vi "PWM Read Duty.vi"(7 "GPIO #":T1=-1, 8 "error in (no error)":errorcluster, 11 "Session in":refnum<class "Session.lvclass">) -> (0 "error out":errorcluster, 2 "Duty % (0-1)":sgl, 3 "Session out":refnum<class "Session.lvclass">)   [LabVIEW 2024, in "CTI.lvlib" / "Session.lvclass"]
doc: "Returns the current duty cycle (as a range from 0.0 to 1.0) of the PWM output. 0 means the output is completely off while 1 is completely on. Varying the duty cycle can be used for operations like controlling the brightness of an LED."
uses:
  Session.lvclass
  GPIO Number.ctl
  DeviceComms/DeviceComms.lvclass
  CTI.lvlib
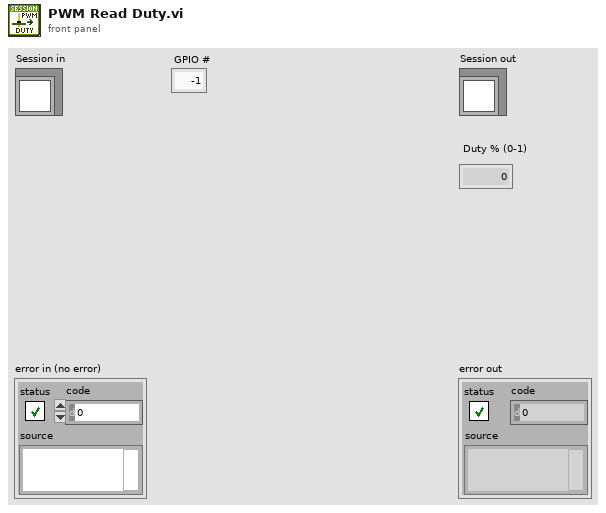
[diagram p1: front panel]
types:
  T1 = typedef "CTI.lvlib/GPIO Number.ctl" = i8
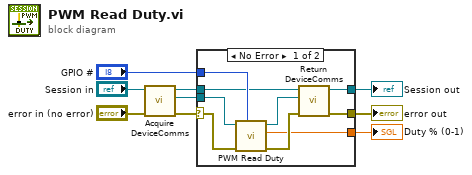
[diagram p0: block diagram]
diagram:
  n1 = call "Acquire DeviceComms.vi"("error in (no error)"="error in (no error)", "Session in"="Session in") -> ("error out"=w8:errorcluster, "DeviceComms"=w7:refnum<class "DeviceComms.lvclass">, "Session out"=w9:refnum<class "Session.lvclass">)  [unwired: 7 in]
  n2 = case shown="No Error" w8 {
    selector: w8 -> [w18 w19]
    tunnel: w9 -> [w15 w20]
    tunnel: w7 -> [w17 _]
    tunnel: "GPIO #" -> [w16 _]
    tunnel: [w12 w19] -> w1
    tunnel: [w11 w20] -> w2
    tunnel: [w10 _] -> w3
    frame No Error {
      n3 = call-dynamic "PWM Read Duty.vi"("GPIO #"=w16, "error in (no error)"=w18, "DeviceComms in"=w17) -> ("error out"=w13:errorcluster, "Duty % (0-1)"=w10:sgl, "DeviceComms out"=w14:refnum<class "DeviceComms.lvclass">)  [unwired: 6 in]
      n4 = call "Return DeviceComms.vi"("error in (no error)"=w13, "DeviceComms"=w14, "Session in"=w15) -> ("error out"=w12:errorcluster, "Session out"=w11:refnum<class "Session.lvclass">)  [unwired: 7 in]
    }
    frame Error {
    }
  }
  "error out" <- w1
  "Session out" <- w2
  "Duty % (0-1)" <- w3
